vi "EMS_Engine_Str.vi"(1 "发送机状态信息":u16(ring) items=["Engine Stop", "Cranking", "Stopping", "Running", "Reserved", "Reserved", "Abnormal", "Invalid"]) -> (0 "CmdStr":string)   [LabVIEW 2013]
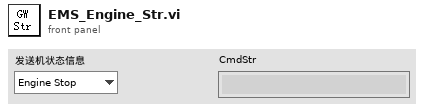
[diagram p1: front panel]
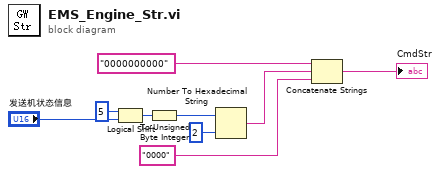
[diagram p0: block diagram]
diagram:
  n1 = Logical Shift(y=5, x="发送机状态信息") -> (x << y=w6:u16)
  n2 = To Unsigned Byte Integer(number=w6) -> (unsigned 8bit integer=w5:u8)
  n3 = Number To Hexadecimal String(1:2, 2:w5) -> (0:w3:string)
  n4 = Concatenate Strings("0000000000", w3, "0000") -> (→"CmdStr":string)
